vi "Position_PID_2.vi"(1 "Target_Position":dbl, 2 "Angle":dbl, 3 "Encoder":dbl) -> (0 "PWM":dbl)   [LabVIEW 2018]
uses:
  Global_variables.vi
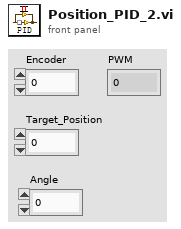
[diagram p1: front panel]
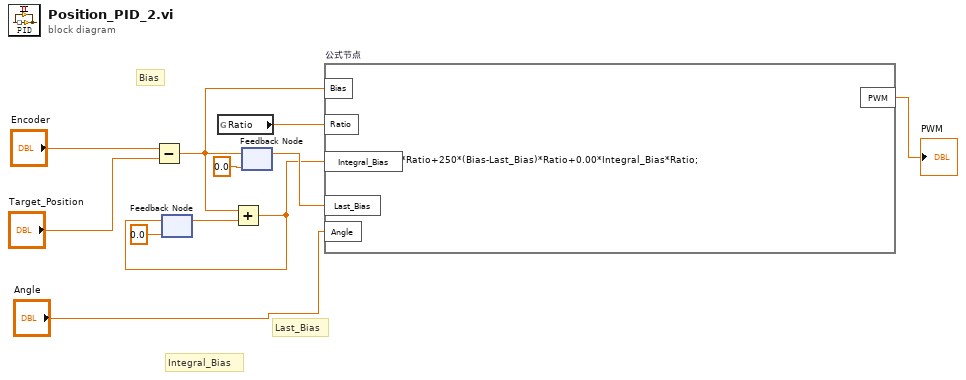
[diagram p0: block diagram]
diagram:
  # "Last_Bias"
  # "Integral_Bias"
  # "Bias"
  n1 = Subtract(x="Encoder", y="Target_Position") -> (x-y=w4:dbl)
  n2 = feedback #1(0.0) -> (w8:dbl)
  n3 = global read "Global_variables.vi" "Ratio"() -> (w3:dbl)
  n4 = Add(x=w4, y=w8) -> (x+y=w5:dbl)
  n5 = feedback-in #1(w5) -> ()
  n6 = feedback-in #2(w4) -> ()
  n7 = feedback #2(0.0) -> (w6:dbl)
  n8 = formula code="PWM=90*Bias*Ratio+250*(Bias-Last_Bias)*Ratio+0.00*Integral_Bias*Ratio;" "公式节点"("Bias"=w4, "Ratio"=w3, "Integral_Bias"=w5, "Last_Bias"=w6, "Angle"="Angle") -> ("PWM"=→"PWM":dbl)
